vi "Two Color Get Connection.vi"(0 "Remote IP":string, 7 "Port":u16, 11 "Error In":errorcluster) -> (4 "Connection ID":refnum<k5>, 8 "Connected?":bool, 15 "Error Out":errorcluster)   [LabVIEW 2020]
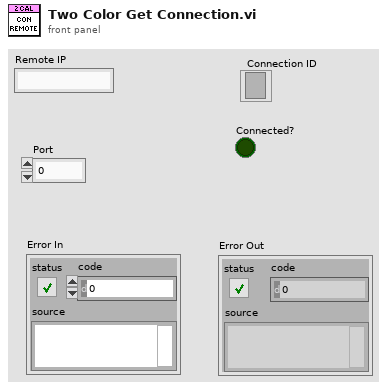
[diagram p1: front panel]
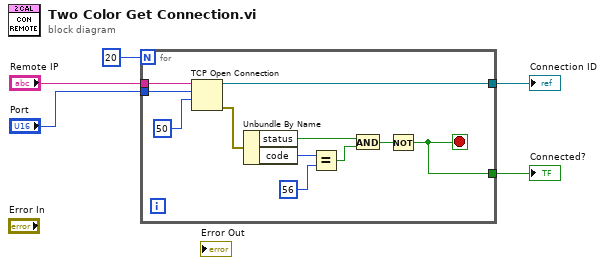
[diagram p0: block diagram]
diagram:
  n1 = for {
    N: 20 -> [_]
    tunnel: "Remote IP" -> [w10]
    tunnel: "Port" -> [w9]
    tunnel: [w7] -> w1
    tunnel: [w6] -> w2
    stop <- w6 stop-if-true
    n2 = TCP Open Connection(address=w10, remote port or service name=w9, timeout ms (60000)=50) -> (connection ID=w7:refnum<k5>, error out=w11:errorcluster)  [unwired: 2 in]
    n3 = Unbundle By Name(w11) -> ("status"=w13:bool, "code"=w16:i32)
    n4 = Equal?(x=w16, y=56) -> (x = y?=w12:bool)
    n5 = And(x=w13, y=w12) -> (x .and. y?=w8:bool)
    n6 = Not(x=w8) -> (.not. x?=w6:bool)
  }
  "Connected?" <- w2
  "Connection ID" <- w1
